vi "tcpListen.vi"() -> ()   [LabVIEW 2021]
panel:
  in  "stop":bool
  out "data out":string
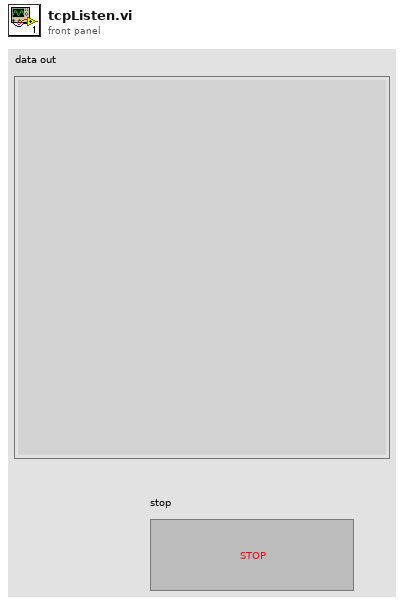
[diagram p1: front panel]
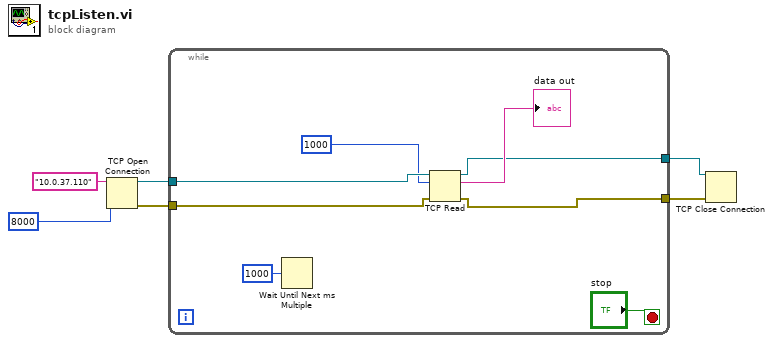
[diagram p0: block diagram]
diagram:
  n1 = TCP Open Connection(address="10.0.37.110", remote port or service name=u16 8000) -> (connection ID=w3:refnum<k5>, error out=w4:errorcluster)  [unwired: 3 in]
  n2 = while {
    tunnel: w4 -> [w13]
    tunnel: w3 -> [w12]
    tunnel: [w11] -> w2
    tunnel: [w10] -> w1
    stop <- "stop" stop-if-true
    n3 = Wait Until Next ms Multiple(millisecond multiple=u32 1000) -> ()  [unwired: 1 out]
    n4 = TCP Read(connection ID=w12, bytes to read=1000, error in (no error)=w13) -> (connection ID out=w10:refnum<k5>, data out=→"data out":string, error out=w11:errorcluster)  [unwired: 2 in]
  }
  n5 = TCP Close Connection(connection ID=w1, error in (no error)=w2) -> ()  [unwired: 1 in, 2 out]
